vi "oa_Search Start and End in Speed Profile.vi"(6 "last value in":cluster{"reference":dbl, "interpolation":dbl}, 7 "reset":bool, 8 "steps input":cluster{"start":dbl, "end":dbl, "step":dbl} {"step" format="%.2f"; "end" format="%.2f"; "start" format="%.2f"}, 9 "next value in":dbl, 10 "interpolation array":dbl[](array[numeric]), 11 "reference array":dbl[](array[numeric])) -> (0 "actual steps":T1 {"step" format="%.2f"; "start" format="%.2f"}, 1 "next value out":dbl, 2 "interpolation array out":dbl[](array[numeric]), 3 "reference array out":dbl[](array[numeric]), 4 "last value out":cluster{"reference":dbl, "interpolation":dbl}, 5 "reach end?":bool)   [LabVIEW 2017]
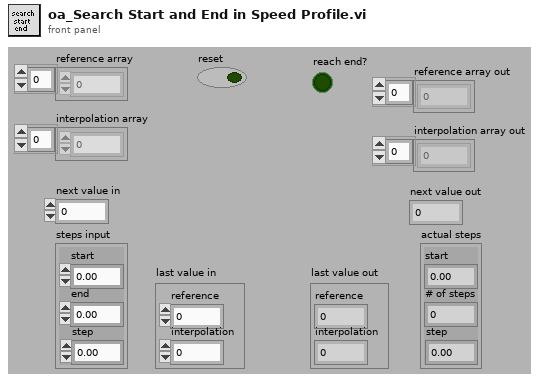
[diagram p1: front panel]
types:
  T1 = cluster{"start":dbl, "# of steps":i32, "step":dbl}
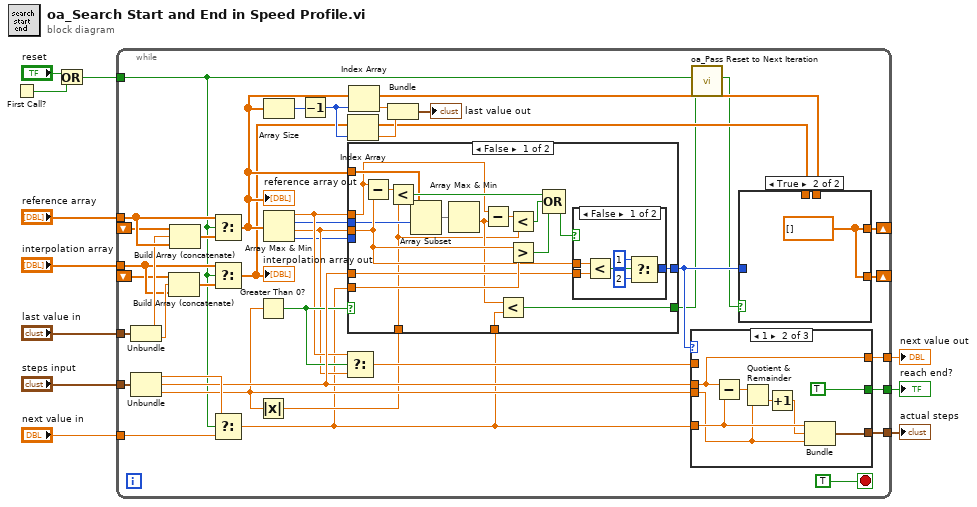
[diagram p0: block diagram]
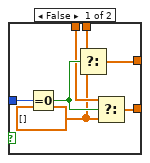
[diagram p2: hidden frame]
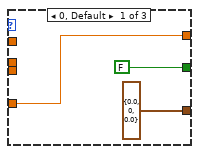
[diagram p3: hidden frame]
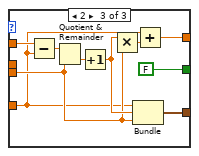
[diagram p4: hidden frame]
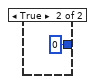
[diagram p5: hidden frame]
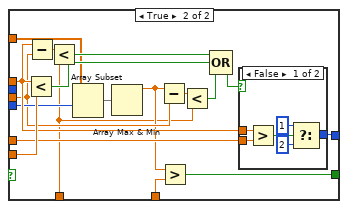
[diagram p6: hidden frame]
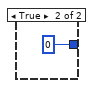
[diagram p7: hidden frame]
diagram:
  n1 = First Call?() -> (First Call?: T/F=w9:bool)
  n2 = Or(x="reset", y=w9) -> (x .or. y?=w5:bool)
  n3 = while {
    tunnel: "steps input" -> [w50]
    tunnel: "next value in" -> [w48]
    tunnel: "last value in" -> [w47]
    tunnel: "reference array" -> [w46]
    tunnel: w5 -> [w15]
    tunnel: "interpolation array" -> [w41]
    tunnel: [w40] -> w3
    tunnel: [w39] -> w2
    tunnel: [w38] -> w1
    shift-right: [w20] -> _
    shift-left: _ -> [w21]
    shift-right: [w18] -> _
    shift-left: _ -> [w17]
    stop <- TRUE stop-if-true
    n4 = Unbundle(w47) -> ("reference"=w45:dbl, "interpolation"=w42:dbl)
    n5 = Unbundle(w50) -> ("start"=w49:dbl, "end"=w32:dbl, "step"=w27:dbl)
    n6 = Build Array (concatenate)(w17, w42, w41) -> (w43:dbl[])
    n7 = Build Array (concatenate)(w21, w45, w46) -> (w44:dbl[])
    n8 = Select(t=w46, s=w15, f=w44) -> (s? t:f=w22:dbl[])
    "reference array out" <- w22
    n9 = Select(t=w41, s=w15, f=w43) -> (s? t:f=w19:dbl[])
    "interpolation array out" <- w19
    n10 = Select(t=w49, s=w15, f=w48) -> (s? t:f=w13:dbl)
    n11 = Greater Than 0?(x=w27) -> (x > 0?=w31:bool)
    n12 = Absolute Value(x=w27) -> (abs(x)=w26:dbl)
    n13 = Array Size(array=w22) -> (size(s)=w37:i32)
    n14 = Array Max & Min(array=w22) -> (max value=w30:dbl, max index (indices)=w25:i32, min value=w29:dbl, min index (indices)=w24:i32)
    n15 = Decrement(x=w37) -> (x-1=w36:i32)
    n16 = Select(t=w30, s=w31, f=w29) -> (s? t:f=w28:dbl)
    n17 = Index Array(array=w19, index=w36) -> (element=w34:dbl)
    n18 = case shown="False" w31 {
      tunnel: w30 -> [w84 w119]
      tunnel: w29 -> [w94 w111]
      tunnel: w13 -> [w97 w122]
      tunnel: w32 -> [w95 w121]
      tunnel: [w96 w120] -> w16
      tunnel: w26 -> [w82 w107]
      tunnel: w25 -> [w87 _]
      tunnel: w24 -> [_ w113]
      tunnel: w22 -> [w88 w114]
      tunnel: [w81 w106] -> w12
      tunnel: w13 -> [w80 w105]
      frame False {
        n19 = Subtract(x=w84, y=w94) -> (x-y=w93:dbl)
        n20 = Less?(x=w93, y=w82) -> (x < y?=w92:bool)
        n21 = Array Subset(array=w88, index=w87) -> (w86:dbl[])  [unwired: 1 in]
        n22 = Array Max & Min(array=w86) -> (min value=w83:dbl)  [unwired: 3 out]
        n23 = Subtract(x=w84, y=w83) -> (x-y=w85:dbl)
        n24 = Less?(x=w83, y=w80) -> (x < y?=w81:bool)
        n25 = Less?(x=w85, y=w82) -> (x < y?=w91:bool)
        n26 = Greater?(x=w94, y=w97) -> (0:w90:bool)
        n27 = Compound Arithmetic op=OR(w92, w91, w90) -> (w89:bool)
        n28 = case shown="False" w89 {
          tunnel: [w99 0] -> w96
          tunnel: w94 -> [w103 _]
          tunnel: w95 -> [w102 _]
          frame False {
            n29 = Less?(x=w103, y=w102) -> (x < y?=w101:bool)
            n30 = Select(t=1, s=w101, f=2) -> (s? t:f=w99:i32)
          }
          frame True {
          }
        }
      }
      frame True {
        n31 = Less?(x=w119, y=w122) -> (x < y?=w116:bool)
        n32 = Subtract(x=w119, y=w111) -> (x-y=w118:dbl)
        n33 = Less?(x=w118, y=w107) -> (x < y?=w117:bool)
        n34 = Array Subset(array=w114, index=w113) -> (w112:dbl[])  [unwired: 1 in]
        n35 = Array Max & Min(array=w112) -> (max value=w108:dbl)  [unwired: 3 out]
        n36 = Subtract(x=w108, y=w111) -> (x-y=w110:dbl)
        n37 = Greater?(x=w108, y=w105) -> (0:w106:bool)
        n38 = Less?(x=w110, y=w107) -> (x < y?=w109:bool)
        n39 = Compound Arithmetic op=OR(w117, w116, w109) -> (w115:bool)
        n40 = case shown="False" w115 {
          tunnel: w119 -> [w128 _]
          tunnel: w121 -> [w127 _]
          tunnel: [w123 0] -> w120
          frame False {
            n41 = Greater?(x=w128, y=w127) -> (0:w126:bool)
            n42 = Select(t=1, s=w126, f=2) -> (s? t:f=w123:i32)
          }
          frame True {
          }
        }
      }
    }
    n43 = Index Array(array=w22, index=w36) -> (element=w35:dbl)
    n44 = Bundle("time [s]"=w35, "speed [rpm]"=w34) -> (→"last value out":cluster{"time [s]":dbl, "speed [rpm]":dbl})  [unwired: 1 in]
    n45 = case shown="1" w16 {
      tunnel: [FALSE ("reach end?") TRUE ("reach end?") FALSE ("reach end?")] -> w40
      tunnel: w13 -> [w60 w68 w71]
      tunnel: [w60 w63 w73] -> w39
      tunnel: [T1 {"start"=0.0, "# of steps"=0, "step"=0.0} ("actual steps") w64 w77] -> w38
      tunnel: w27 -> [_ w66 w75]
      tunnel: w32 -> [_ w63 _]
      tunnel: w28 -> [_ _ w72]
      frame 0, Default {
      }
      frame 1 {
        n46 = Subtract(x=w63, y=w68) -> (x-y=w67:dbl)
        n47 = Quotient & Remainder(x=w67, y=w66) -> (floor(x/y)=w62:dbl)  [unwired: 1 out]
        n48 = Increment(x=w62) -> (x+1=w65:dbl)
        n49 = Bundle("next value in"=w68, w65, "step"=w66) -> (w64:cluster{"next value in":dbl, dbl, "step":dbl})  [unwired: 1 in]
      }
      frame 2 {
        n50 = Subtract(x=w72, y=w71) -> (x-y=w78:dbl)
        n51 = Quotient & Remainder(x=w78, y=w75) -> (floor(x/y)=w70:dbl)  [unwired: 1 out]
        n52 = Increment(x=w70) -> (x+1=w76:dbl)
        n53 = Multiply(x=w76, y=w75) -> (x*y=w74:dbl)
        n54 = Bundle("next value in"=w71, w76, "step"=w75) -> (w77:cluster{"next value in":dbl, dbl, "step":dbl})  [unwired: 1 in]
        n55 = Add(x=w71, y=w74) -> (x+y=w73:dbl)
      }
    }
    n56 = call <vilib>:"oa_Pass Reset to Next Iteration.vi"("trigger"=w12, "reset?(F)"=w15) -> ("reset out"=w14:bool)  [unwired: 9 in]
    n57 = case shown="True" w14 {
      tunnel: w16 -> [w57 _]
      tunnel: w22 -> [w56 _]
      tunnel: [w55 w58] -> w20
      tunnel: w19 -> [w53 _]
      tunnel: [w51 w58] -> w18
      frame False {
        w52 = dbl[] [] ("f")
        n58 = Equal To 0?(x=w57) -> (x = 0?=w54:bool)
        n59 = Select(t=w56, s=w54, f=w52) -> (s? t:f=w55:dbl[])
        n60 = Select(t=w53, s=w54, f=w52) -> (s? t:f=w51:dbl[])
      }
      frame True {
        w58 = dbl[] [] ("f")
      }
    }
  }
  "next value out" <- w2
  "reach end?" <- w3
  "actual steps" <- w1
